vi "Read.vi"(8 "error in (no error)":errorcluster, 11 "Cluster Array in":refnum<class "Cluster Array.lvclass">) -> (0 "error out":errorcluster, 2 "Cluster Array":refnum<class "Cluster.lvclass">[](array[class]), 3 "Cluster Array out":refnum<class "Cluster Array.lvclass">)   [LabVIEW 2020, in "Data.lvlib" / "Cluster Array.lvclass"]
doc: "Read Cluster Array."
uses:
  Cluster Array.lvclass
  Cluster/Cluster.lvclass
  Cluster Array.lvclass/Cluster Array.ctl
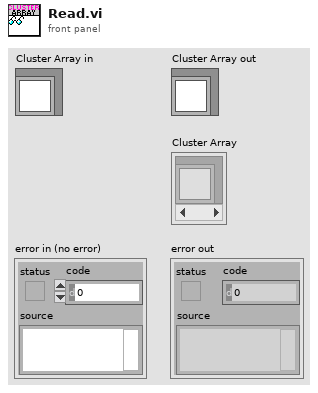
[diagram p1: front panel]
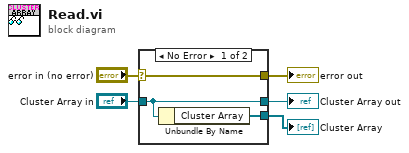
[diagram p0: block diagram]
diagram:
  n1 = case shown="No Error" "error in (no error)" {
    selector: "error in (no error)" -> [w8 w9]
    tunnel: [w8 w9] -> w4
    tunnel: [w7 w10] -> w2
    tunnel: "Cluster Array in" -> [w7 w10]
    tunnel: [w6 _] -> w1
    frame No Error {
      n2 = Unbundle By Name(w7) -> ("Cluster Array"=w6:refnum<class "Cluster.lvclass">[])
    }
    frame Error {
    }
  }
  "error out" <- w4
  "Cluster Array out" <- w2
  "Cluster Array" <- w1
